vi "Wait for Server.vi"(0 "error in":errorcluster, 2 "vi reference in":refnum<vi>) -> (1 "error out":errorcluster, 3 "Error?":bool, 4 "vi reference out":refnum<vi>)   [LabVIEW 2013]
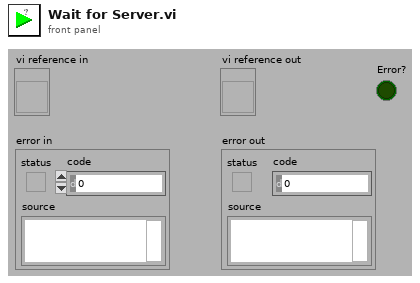
[diagram p1: front panel]
types:
  T1 = enum32{"Bad", "Idle", "Run top level", "Running"}
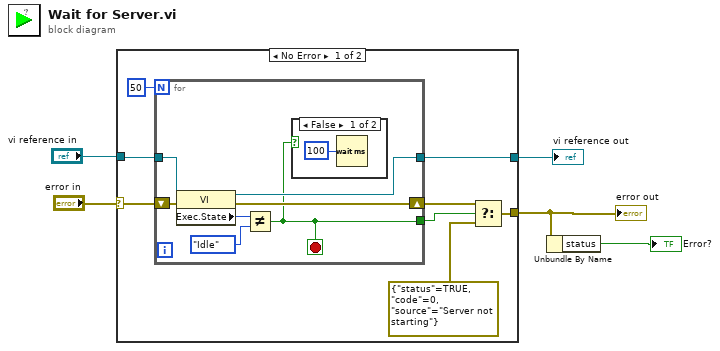
[diagram p0: block diagram]
diagram:
  n1 = case shown="No Error" "error in" {
    selector: "error in" -> [w6 w22]
    tunnel: "vi reference in" -> [w12 w23]
    tunnel: [w11 w23] -> w4
    tunnel: [w8 w22] -> w2
    frame No Error {
      n2 = for {
        N: 50 -> [_]
        tunnel: w12 -> [w20]
        shift-right: [w16] -> w9
        shift-left: w6 -> [w17]
        tunnel: [w15] -> w11
        tunnel: [w14] -> w10
        stop <- w14 stop-if-true
        n3 = property class="VI"(reference=w20, error in=w17) -> (reference out=w15:refnum<vi>, error out=w16:errorcluster, "Exec.State"=w19:T1)
        n4 = Not Equal?(x=w19, y=T1."Idle") -> (x != y?=w14:bool)
        n5 = case shown="False" w14 {
          frame False {
            n6 = Wait (ms)(milliseconds to wait=u32 100) -> ()  [unwired: 1 out]
          }
          frame True {
          }
        }
      }
      n7 = Select(t=w9, s=w10, f=errorcluster {"status"=TRUE, "code"=0, "source"="Server not starting"}) -> (s? t:f=w8:errorcluster)
    }
    frame Error {
    }
  }
  "vi reference out" <- w4
  "error out" <- w2
  n8 = Unbundle By Name(w2) -> ("status"=→"Error?":bool)
